vi "PH_BlackBox.set GUI Refs.vi"(0 "VI in":refnum<vi>, 2 "GUI Refs":T1, 5 "error in (no error)":errorcluster) -> (14 "VI out":refnum<vi>, 19 "error out":errorcluster)   [LabVIEW 2014, in "PH_BlackBox.lvlib"]
uses:
  PH_BlackBox.lvlib
  PH_BlackBox.GUI Refs.ctl
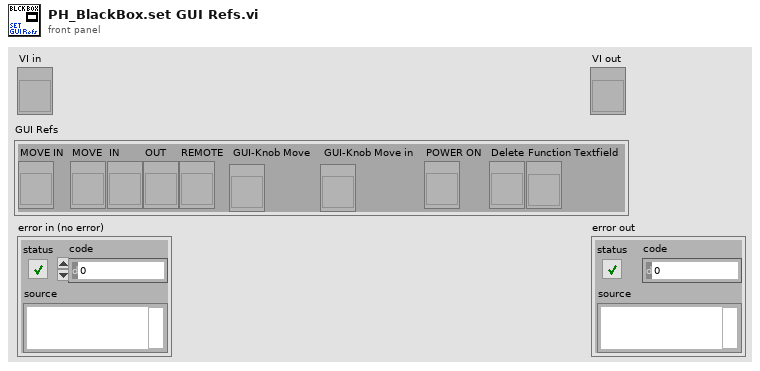
[diagram p1: front panel]
types:
  T1 = typedef "PH_BlackBox.lvlib/PH_BlackBox.GUI Refs.ctl" = cluster{"MOVE IN":refnum<vi>, "MOVE":refnum<vi>, "IN":refnum<vi>, "OUT":refnum<vi>, "REMOTE":refnum<vi>, "GUI-Knob Move":refnum<vi>, "GUI-Knob Move in":refnum<vi>, "POWER ON":refnum<vi>, "Delete":refnum<vi>, "Function Textfield":refnum<vi>}
  T2 = typedef "PH_BlackBox.lvlib/PH_BlackBox.i attribute.ctl" = cluster{"BB Remote Controlled?":bool, "GUI Refs":T1, "Position IN":T3, "Position OUT":T3, "BB Remote Controlled by other Instance?":bool, "Recipient":string, "Number":i32, "Caption Move":string, "Caption Out":string, "Caption In":string}
  T3 = typedef "PH_StatusHandler.lvlib/PH_StatusHandler.Status.ctl" = i16
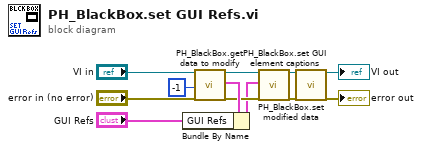
[diagram p0: block diagram]
diagram:
  n1 = call "PH_BlackBox.get data to modify.vi"("i ref in"="VI in", "ms timeout (10000)"=-1, "error in (no error)"="error in (no error)") -> ("i ref out"=w7:refnum<vi>, "i attribute"=w12:T2, "error out"=w8:errorcluster)  [unwired: 13 in, 1 out]
  n2 = Bundle By Name(cluster=w12, "GUI Refs"="GUI Refs") -> (w4:T2)
  n3 = call "PH_BlackBox.set modified data.vi"("i ref in"=w7, "i attribute"=w4, "error in (no error)"=w8) -> ("i ref out"=w6:refnum<vi>, "error out"=w5:errorcluster)  [unwired: 15 in]
  n4 = call "PH_BlackBox.set GUI element captions.vi"("i ref in"=w6, "error in (no error)"=w5) -> ("i ref out"=→"VI out":refnum<vi>, "error out"=→"error out":errorcluster)  [unwired: 16 in]
